vi "moveBlockDiagramFlatSequence.vi"(8 "error in":errorcluster caption="에러 입력", 9 "대상객체":string, 10 "목표위치":string, 11 "VI 참조":refnum<vi>) -> (0 "error out":errorcluster caption="에러 출력", 3 "성공?":bool)   [LabVIEW 2018]
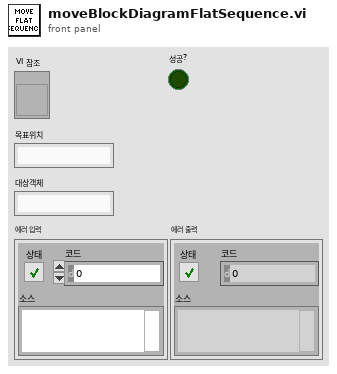
[diagram p1: front panel]
types:
  T1 = typedef "LVPositionTypeDef.ctl" = cluster{"Left":i32, "Top":i32}
  T2 = cluster{"Label.Text":string, refnum<vi>, "Position":T1}
  T3 = cluster{"Label.Text":string, refnum<vi>, "Position":T1}[]
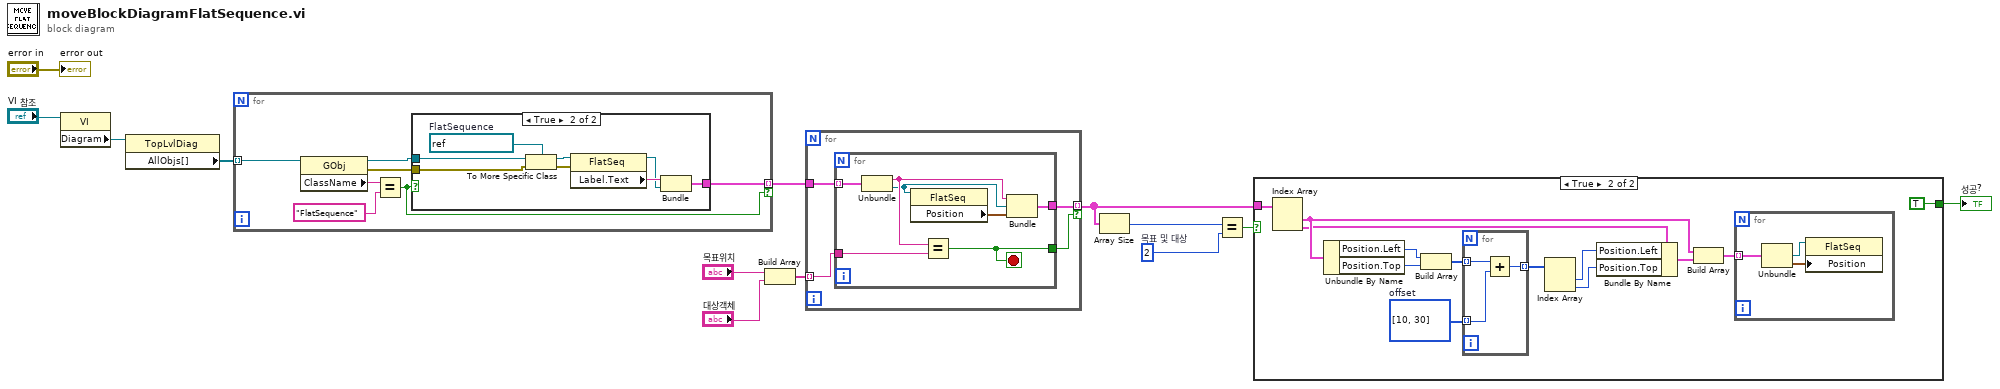
[diagram p0: block diagram]
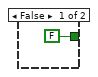
[diagram p2: hidden frame]
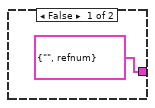
[diagram p3: hidden frame]
diagram:
  w5 = 2  # 목표 및 대상
  n1 = property class="VI"(reference="VI 참조") -> ("Diagram"=w12:refnum<vi>)  [unwired: 1 in, 2 out]
  n2 = property class="TopLvlDiag"(reference=w12) -> ("AllObjs[]"=w13:refnum<vi>[])  [unwired: 1 in, 2 out]
  n3 = for {
    tunnel: w13 -> [w20] mode=indexing
    tunnel: [w14] -> w2 mode=indexing if=w16
    n4 = property class="GObj"(reference=w20) -> (reference out=w15:refnum<vi>, error out=w19:errorcluster, "ClassName"=w18:string)  [unwired: 1 in]
    n5 = Equal?(x=w18, y="FlatSequence") -> (x = y?=w16:bool)
    n6 = case shown="True" w16 {
      tunnel: w15 -> [_ w29]
      tunnel: w19 -> [_ w28]
      tunnel: [cluster{string, refnum<vi>} {"", refnum} w22] -> w14
      frame False {
      }
      frame True {
        w27 = refnum<vi> refnum  # FlatSequence
        n7 = To More Specific Class(target class=w27, reference=w29, error in=w28) -> (specific class reference=w26:refnum<vi>, error out=w25:errorcluster)
        n8 = property class="FlatSeq"(reference=w26, error in=w25) -> (reference out=w23:refnum<vi>, "Label.Text"=w24:string)  [unwired: 1 out]
        n9 = Bundle("Label.Text"=w24, w23) -> (w22:cluster{"Label.Text":string, refnum<vi>})  [unwired: 1 in]
      }
    }
  }
  n10 = Build Array("목표위치", "대상객체") -> (w7:string[])
  n11 = for {
    tunnel: w2 -> [w33]
    tunnel: w7 -> [w32] mode=indexing
    tunnel: [w30] -> w3 mode=indexing if=w31
    n12 = for {
      tunnel: w33 -> [w40] mode=indexing
      tunnel: w32 -> [w39]
      tunnel: [w38] -> w31
      tunnel: [w34] -> w30
      stop <- w38 stop-if-true
      n13 = Unbundle(w40) -> ("Label.Text"=w37:string, w36:refnum<vi>)
      n14 = property class="FlatSeq"(reference=w36) -> ("Position"=w35:T1)  [unwired: 1 in, 2 out]
      n15 = Equal?(x=w37, y=w39) -> (x = y?=w38:bool)
      n16 = Bundle("Label.Text"=w37, w36, "Position"=w35) -> (w34:T2)  [unwired: 1 in]
    }
  }
  n17 = Array Size(array=w3) -> (size(s)=w6:i32)
  n18 = Equal?(x=w6, y=w5) -> (x = y?=w4:bool)
  n19 = case shown="True" w4 {
    tunnel: w3 -> [_ w49]
    tunnel: [FALSE TRUE] -> w1
    frame False {
    }
    frame True {
      w42 = i32[] [10, 30]  # offset
      n20 = Index Array(array=w49) -> (element #1=w54:T2, element #2=w53:T2)  [unwired: 2 in]
      n21 = Unbundle By Name(w54) -> ("Position.Left"=w48:i32, "Position.Top"=w47:i32)
      n22 = Build Array(w48, w47) -> (w46:i32[])
      n23 = for {
        tunnel: w46 -> [w57] mode=indexing
        tunnel: [w56] -> w45 mode=indexing
        tunnel: w42 -> [w55] mode=indexing
        n24 = Add(x=w57, y=w55) -> (x+y=w56:i32)
      }
      n25 = Index Array(array=w45) -> (element #1=w44:i32, element #2=w43:i32)  [unwired: 2 in]
      n26 = Bundle By Name(cluster=w53, "Position.Left"=w44, "Position.Top"=w43) -> (w52:T2)
      n27 = Build Array(w54, w52) -> (w51:T3)
      n28 = for {
        tunnel: w51 -> [w60] mode=indexing
        n29 = Unbundle(w60) -> (w58:refnum<vi>, "Position"=w59:T1)  [unwired: 1 out]
        n30 = property class="FlatSeq"(reference=w58, "Position"=w59) -> ()  [unwired: 1 in, 2 out]
      }
    }
  }
  "성공?" <- w1
  "error out" <- "error in"
